vi "Write Digital Output.vi"(8 "error in (no error)":errorcluster, 10 "Digital Output":T1(array[cluster]) {"expiration state" items=["High"=10192, "Low"=10214, "Tristate"=10310, "No Change"=10160]}, 11 "DAQmx Watchdog configuration in":refnum<class "DAQmx Watchdog configuration.lvclass">) -> (0 "error out":errorcluster, 3 "DAQmx Watchdog configuration out":refnum<class "DAQmx Watchdog configuration.lvclass">)   [LabVIEW 2014, in "DAQmx Watchdog configuration.lvclass"]
uses:
  DAQmx Watchdog configuration.lvclass
  DAQmx Watchdog configuration.lvclass/DAQmx Watchdog configuration.ctl
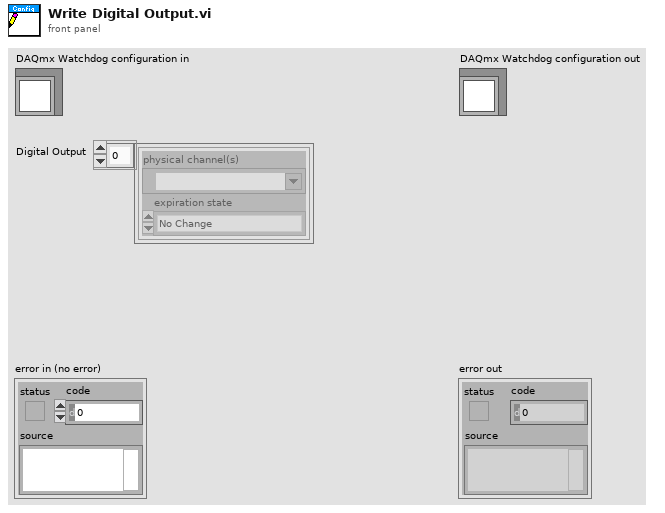
[diagram p1: front panel]
types:
  T1 = cluster{"physical channel(s)":tag, "expiration state":i32}[]
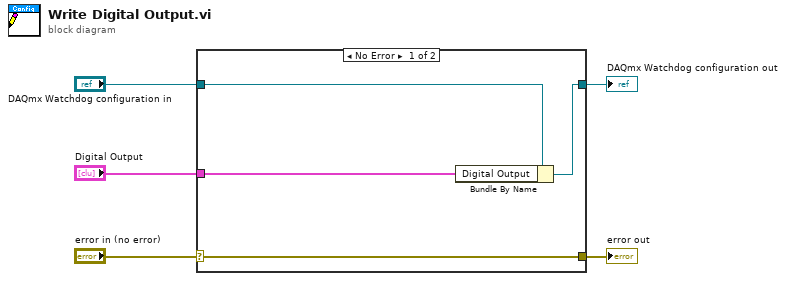
[diagram p0: block diagram]
diagram:
  n1 = case shown="No Error" "error in (no error)" {
    selector: "error in (no error)" -> [w9 w10]
    tunnel: [w9 w10] -> w4
    tunnel: [w7 w11] -> w2
    tunnel: "DAQmx Watchdog configuration in" -> [w8 w11]
    tunnel: "Digital Output" -> [w6 _]
    frame No Error {
      n2 = Bundle By Name(cluster=w8, "Digital Output"=w6) -> (w7:refnum<class "DAQmx Watchdog configuration.lvclass">)
    }
    frame Error {
    }
  }
  "error out" <- w4
  "DAQmx Watchdog configuration out" <- w2
